vi "counter.vi"() -> ()   [LabVIEW 2014]
panel:
  out "counter":dbl
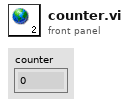
[diagram p1: front panel]
diagram:
